vi "Read Valve Parameters.vi"(7 "listen period":sgl=0.1, 8 "error in":errorcluster, 11 "Brooks MFC in":refnum<class "Brooks MFC.lvclass">) -> (0 "error out":errorcluster, 1 "Valve Range":i32=5391, 2 "Valve Offset":i32=13225, 3 "Brooks MFC out":refnum<class "Brooks MFC.lvclass">)   [LabVIEW 2016, in "Brooks MFC.lvclass"]
uses:
  Brooks MFC.lvclass
  Brooks MFC.lvclass/Brooks MFC.ctl
  Instance           4 29Saved   Read Valve Parameters .vi
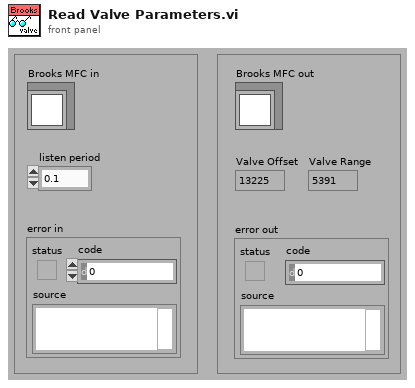
[diagram p1: front panel]
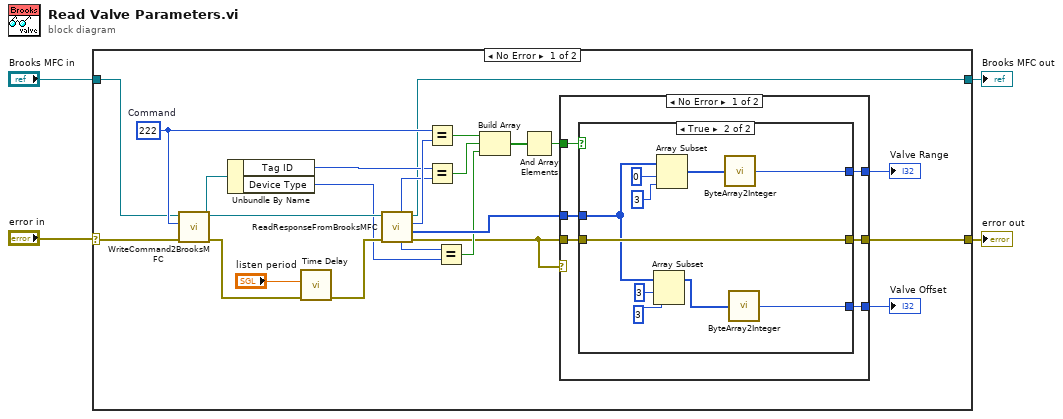
[diagram p0: block diagram]
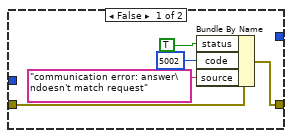
[diagram p2: hidden frame]
diagram:
  n1 = case shown="No Error" "error in" {
    selector: "error in" -> [w6 w50]
    tunnel: "Brooks MFC in" -> [w11 w51]
    tunnel: [w7 w51] -> w2
    tunnel: [w5 w50] -> w1
    frame No Error {
      w13 = u8 222  # Command
      n2 = call "WriteCommand2BrooksMFC.vi"("error in"=w6, "Command"=w13, "Brooks MFC in"=w11) -> ("error out"=w23:errorcluster, "Brooks MFC out"=w10:refnum<class "Brooks MFC.lvclass">)  [unwired: 6 in, 1 out]
      n3 = Unbundle By Name(w10) -> ("Tag ID"=w8:u32, "Device Type"=w9:u8)
      n4 = call "Time Delay"("error in (no error)"=w23, "Delay Time (s)"="listen period") -> ("error out"=w22:errorcluster)  [unwired: 9 in]
      n5 = call "ReadResponseFromBrooksMFC.vi"("error in"=w22, "Brooks MFC in"=w10) -> ("error out"=w12:errorcluster, "Data"=w27:u8[], "Command"=w24:u8, "Brooks MFC out"=w7:refnum<class "Brooks MFC.lvclass">, "device type"=w17:u8, "tag ID"=w16:u32)  [unwired: 4 in]
      n6 = Equal?(x=w13, y=w24) -> (x = y?=w20:bool)
      n7 = Equal?(x=w8, y=w16) -> (x = y?=w14:bool)
      n8 = Equal?(x=w17, y=w9) -> (x = y?=w15:bool)
      n9 = Build Array(w20, w14, w15) -> (w19:bool[])
      n10 = And Array Elements(Boolean array=w19) -> (logical AND=w18:bool)
      n11 = case shown="No Error" w12 {
        tunnel: w12 -> [w33 w49]
        tunnel: w27 -> [w32 _]
        tunnel: [w31 w49] -> w5
        tunnel: [w30 _] -> w26
        tunnel: [w29 _] -> w25
        tunnel: w18 -> [w28 _]
        frame No Error {
          n12 = case shown="True" w28 {
            tunnel: w32 -> [_ w45]
            tunnel: w33 -> [w36 w46]
            tunnel: [w35 w46] -> w31
            tunnel: [_ w40] -> w30
            tunnel: [_ w41] -> w29
            frame False {
              n13 = Bundle By Name(cluster=w36, "status"=TRUE ("Bundle Element"), "code"=5002 ("Bundle Element"), "source"="communication error: answer\ndoesn't match request") -> (w35:errorcluster)
            }
            frame True {
              n14 = Array Subset(array=w45, index=3 ("Array Index"), length=3 ("Array Length")) -> (w39:u8[])
              n15 = Array Subset(array=w45, index=0 ("Index"), length=3) -> (w42:u8[])
              n16 = call "ByteArray2Integer.vi"("Byte Array"=w42) -> ("Integer"=w41:u32)
              n17 = call "ByteArray2Integer.vi"("Byte Array"=w39) -> ("Integer"=w40:u32)
            }
          }
        }
        frame Error {
        }
      }
      "Valve Range" <- w25
      "Valve Offset" <- w26
    }
    frame Error {
    }
  }
  "Brooks MFC out" <- w2
  "error out" <- w1
